vi "Read message.vi"(8 "error in (no error)":errorcluster, 11 "Messenger in":refnum<class "Messenger.lvclass">) -> (0 "error out":errorcluster, 1 "new msg":bool, 2 "message":string, 3 "Messenger out":refnum<class "Messenger.lvclass">)   [LabVIEW 2018]
uses:
  Messenger.lvclass
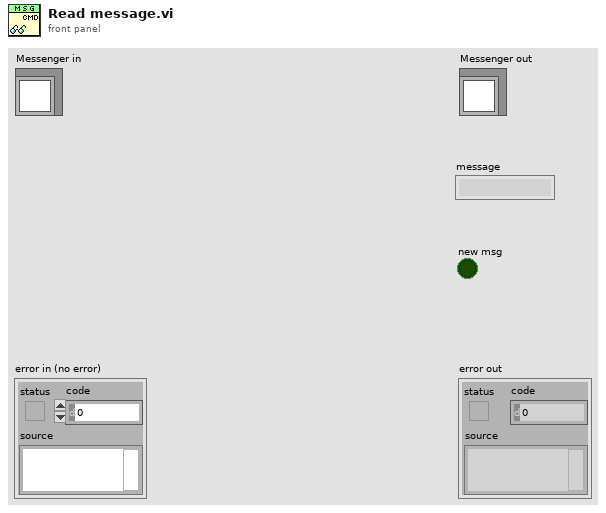
[diagram p1: front panel]
types:
  T1 = typedef "Message Queue.lvlib/Message Cluster.ctl" = cluster{"Message":string, "Message Data":variant}
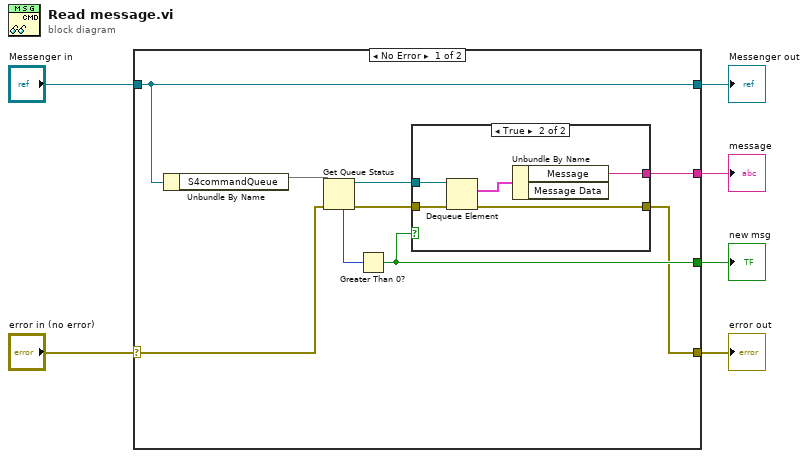
[diagram p0: block diagram]
diagram:
  n1 = case shown="No Error" "error in (no error)" {
    selector: "error in (no error)" -> [w13 w22]
    tunnel: [w7 w22] -> w5
    tunnel: [w15 w23] -> w3
    tunnel: "Messenger in" -> [w15 w23]
    tunnel: [w9 _] -> w2
    tunnel: [w8 _] -> w1
    frame No Error {
      n2 = Unbundle By Name(w15) -> ("S4commandQueue"=w14)
      n3 = Get Queue Status(queue=w14, error in (no error)=w13) -> (queue out=w10:refnum<queue>, error out=w11:errorcluster, # elements in queue=w12:i32)  [unwired: 1 in, 5 out]
      n4 = Greater Than 0?(x=w12) -> (x > 0?=w9:bool)
      n5 = case shown="True" w9 {
        tunnel: w11 -> [w16 w21]
        tunnel: w10 -> [_ w20]
        tunnel: [_ w18] -> w8
        tunnel: [w16 w17] -> w7
        frame False {
        }
        frame True {
          n6 = Dequeue Element(queue=w20, error in (no error)=w21) -> (element=w19:T1, error out=w17:errorcluster)  [unwired: 1 in, 2 out]
          n7 = Unbundle By Name(w19) -> ("Message"=w18:string)  [unwired: 1 out]
        }
      }
    }
    frame Error {
    }
  }
  "error out" <- w5
  "Messenger out" <- w3
  "new msg" <- w2
  "message" <- w1
